vi "IsTransitionComplete.vi"(6 "Last Commanded Regime":T1, 7 "Altered regime boundaries":T2=[0, 70, 140, 220, 190, 360], 8 "Current Regime":T1, 9 "Desired Regime":T1, 10 "Desired Heading (deg)":dbl, 11 "Robot Heading (deg)":dbl) -> (3 "Is Transition Complete?":bool)   [LabVIEW 2013]
doc: "This VI should check whether the boat's current transition is complete, and should probably do so by comparing the desired heading to the boat's actual heading. Once the two are within some error bound, this VI returns 'TRUE' and tells the boat the turn is over.\n\nIf the commanded regime is not adjacent to the desired regime (e.g. we are tacking but we want to end in the reach regime, not the upwind regime) then this VI considers the center of the upwind regime as the new desired heading and checks off the tack transition. At that boat the code above this should say \"I'm in Upwind and want to be reaching, I'm going to command the next transition state\". This way the boat will switch transition states as it goes around the circle seen in https://docs.google.com/file/d/0B6St7IDGiYunU3FLWTZHTUFHWHc/edit?usp=drive_web\n\nEric Schneider, Feb. 2014"
uses:
  Data/TypeDefs/Sailing Regimes.ctl
  Data/TypeDefs/Regime Boundaries.ctl
  Utilities/Math/Angles/Angle/Angle.lvclass
panel:
  in  "Cutoff Range For Completion (deg)":i32=10
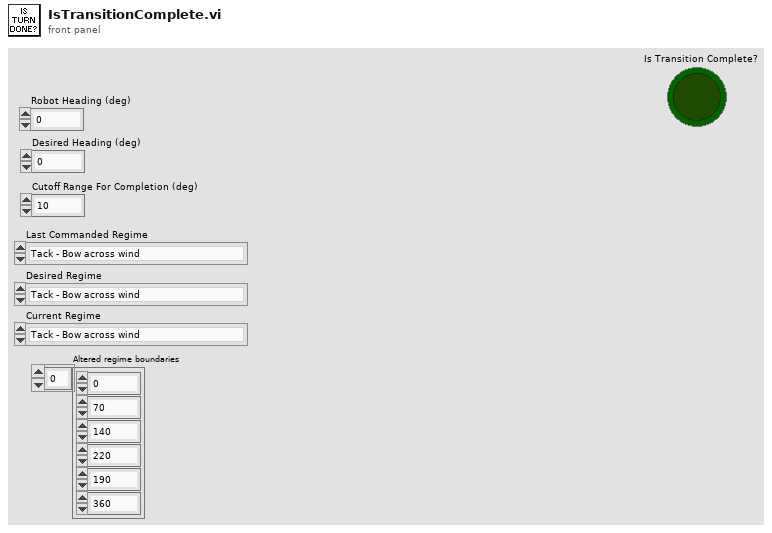
[diagram p1: front panel]
types:
  T1 = typedef "Sailing Regimes.ctl" = enum16{"Tack - Bow across wind", "Upwind - Starboard Tack", "Turn between Upwind/Reach - Starboard Tack", "Reach - Starboard Tack", "Turn between Reach/Run - Starboard Tack", "Run - Starboard Tack", "Jibe - Stern across wind", "Run - Port Tack", "Turn between Reach/Run - Port Tack", "Reach - Port Tack", "Turn between Upwind/Reach - Port Tack", "Upwind - Port Tack"}
  T2 = typedef "Regime Boundaries.ctl" = i32[]
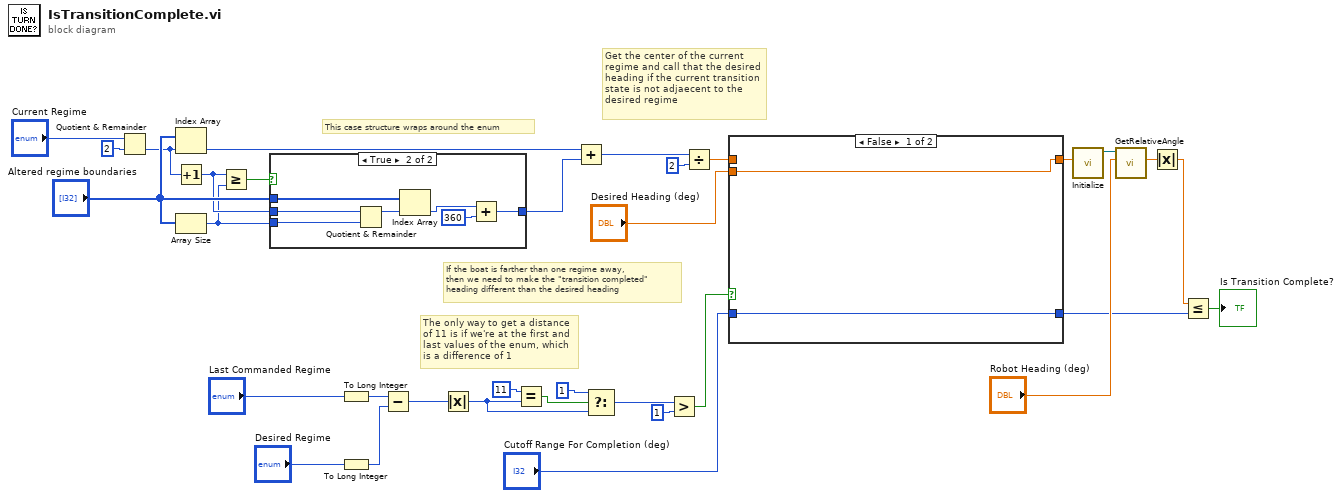
[diagram p0: block diagram]
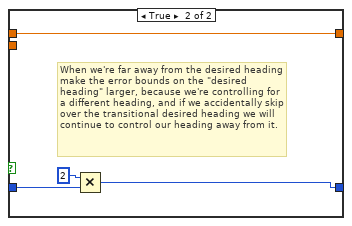
[diagram p2: hidden frame]
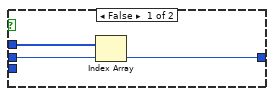
[diagram p3: hidden frame]
diagram:
  # "The only way to get a distance of 11 is if we're at the first and last values of the enum, which is a difference of 1"
  # "This case structure wraps around the enum"
  # "Get the center of the current regime and call that the desired heading if the current transition state is not adjaecent to the desired regime"
  # "If the boat is farther than one regime away,\nthen we need to make the \"transition completed\"\nheading different than the desired heading"
  n1 = Quotient & Remainder(x="Current Regime", y=2) -> (floor(x/y)=w19:i32)  [unwired: 1 out]
  n2 = Index Array(array="Altered regime boundaries", index=w19) -> (element=w13:i32)
  n3 = Increment(x=w19) -> (x+1=w17:i32)
  n4 = Array Size(array="Altered regime boundaries") -> (size(s)=w16:i32)
  n5 = Greater Or Equal?(x=w17, y=w16) -> (x >= y?=w18:bool)
  n6 = case shown="True" w18 {
    tunnel: "Altered regime boundaries" -> [w36 w43]
    tunnel: w17 -> [w35 w41]
    tunnel: w16 -> [_ w40]
    tunnel: [w34 w37] -> w14
    frame False {
      n7 = Index Array(array=w36, index=w35) -> (element=w34:i32)
    }
    frame True {
      n8 = Quotient & Remainder(x=w41, y=w40) -> (x-y*floor(x/y)=w39:i32)  [unwired: 1 out]
      n9 = Index Array(array=w43, index=w39) -> (element=w42:i32)
      n10 = Add(x=w42, y=360) -> (x+y=w37:i32)
    }
  }
  n11 = To Long Integer(number="Last Commanded Regime") -> (32bit integer=w28:i32)
  n12 = To Long Integer(number="Desired Regime") -> (32bit integer=w26:i32)
  n13 = Subtract(x=w28, y=w26) -> (x-y=w25:i32)
  n14 = Absolute Value(x=w25) -> (abs(x)=w4:i32)
  n15 = Equal?(x=11, y=w4) -> (x = y?=w2:bool)
  n16 = Add(x=w13, y=w14) -> (x+y=w15:i32)
  n17 = Select(t=1, s=w2, f=w4) -> (s? t:f=w3:i32)
  n18 = Greater?(x=w3, y=1) -> (0:w11:bool)
  n19 = Divide(x=w15, y=2) -> (x/y=w8:dbl)
  n20 = case shown="False" w11 {
    tunnel: "Desired Heading (deg)" -> [w45 _]
    tunnel: [w45 w49] -> w9
    tunnel: w8 -> [_ w49]
    tunnel: "Cutoff Range For Completion (deg)" -> [w44 w48]
    tunnel: [w44 w46] -> w6
    frame False {
    }
    frame True {
      # "When we're far away from the desired heading make the error bounds on the \"desired heading\" larger, because we're controlling for a different heading, and if we accidentally skip over the transitional desired heading we will continue to control our heading away from it."
      n21 = Multiply(x=2, y=w48) -> (x*y=w46:i32)
    }
  }
  n22 = call "Initialize.vi"("Input Angle (Deg.)"=w9) -> ("Angle out"=w33:refnum<class "Angle.lvclass">)  [unwired: 9 in, 1 out]
  n23 = call "GetRelativeAngle.vi"("Boat Heading (Deg.)"="Robot Heading (deg)", "Angle in"=w33) -> ("Relative Angle"=w31:dbl)  [unwired: 8 in, 1 out]
  n24 = Absolute Value(x=w31) -> (abs(x)=w30:dbl)
  n25 = Less Or Equal?(x=w30, y=w6) -> (x <= y?=→"Is Transition Complete?":bool)
